vi "Far--L.vi"(6 "Command Info In":T2, 8 "Far--L":T1={"1a"=0.0, "1d"=100.5, "1s"=0.8}) -> (0 "Command Info Out":T2)   [LabVIEW 2017]
uses:
  <vilib>/Rock Robotics/WPI/Framework/Command Status Info.ctl
  <vilib>/Rock Robotics/WPI/Framework/Completion Status.ctl
  <vilib>/Rock Robotics/WPI/Framework/Completion Notifier.ctl
  Block Clusters/Far--L.ctl
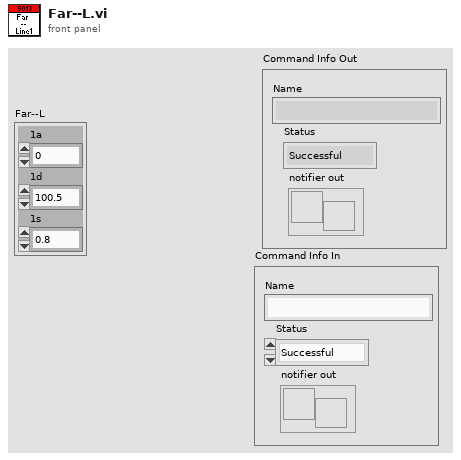
[diagram p1: front panel]
types:
  T1 = typedef "Far--L.ctl" = cluster{"1a":dbl, "1d":dbl, "1s":dbl}
  T2 = typedef "Command Status Info.ctl" = cluster{"Name":string, "Status":T3, "notifier out":T4}
  T3 = typedef "Completion Status.ctl" = enum16{"Successful", "Aborted", "Incomplete"}
  T4 = typedef "Completion Notifier.ctl" = refnum<notifier>
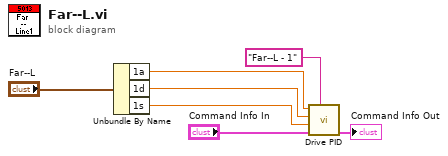
[diagram p0: block diagram]
diagram:
  n1 = Unbundle By Name("Far--L") -> ("1a"=w2:dbl, "1d"=w4:dbl, "1s"=w3:dbl)
  n2 = call "Drive PID.vi"("Description"="Far--L - 1", "Command Info In"="Command Info In", "Speed"=w3, "Distance"=w4, "Target Angle"=w2) -> ("Command Info Out"=→"Command Info Out":T2)  [unwired: 6 in]
